vi "Calculate_Release_Flowrates.vi"(3 "Ch names":string[](array[string]), 4 "Units":enum16{"Q l/min", "M_dot Kg/min"}(ring), 5 "Present scan array":dbl[](array[numeric]) format="%.2f") -> (0 "Trace":dbl format="%.2f", 1 "Carrier":dbl format="%.2f", 2 "Scan comments":string)   [LabVIEW 2015]
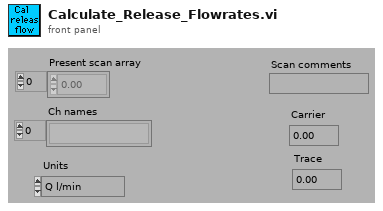
[diagram p1: front panel]
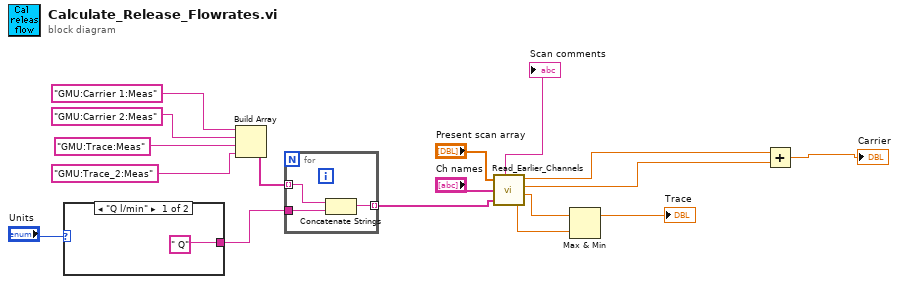
[diagram p0: block diagram]
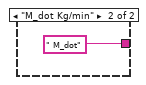
[diagram p2: hidden frame]
diagram:
  n1 = case shown="\"Q l/min\"" "Units" {
    tunnel: [" Q" " M_dot"] -> w16
    frame "Q l/min" {
    }
    frame "M_dot Kg/min" {
    }
  }
  n2 = Build Array("GMU:Carrier 1:Meas", "GMU:Carrier 2:Meas", "GMU:Trace:Meas", "GMU:Trace_2:Meas") -> (w15:string[])
  n3 = for {
    tunnel: w16 -> [w22]
    tunnel: w15 -> [w21] mode=indexing
    tunnel: [w20] -> w7 mode=indexing
    n4 = Concatenate Strings(w21, w22) -> (w20:string)
  }
  n5 = call "Read_Earlier_Channels.vi"("Present scan array"="Present scan array", "Ch names"="Ch names", "Desired Channels"=w7) -> ("Scan comments"=→"Scan comments":string, "Index 0"=w6:dbl, "Index 1"=w5:dbl, "Index 2"=w3:dbl, "Index 3"=w2:dbl)  [unwired: 1 out]
  n6 = Max & Min(x=w3, y=w2) -> (max(x,y)=→"Trace":dbl)  [unwired: 1 out]
  n7 = Add(x=w6, y=w5) -> (x+y=→"Carrier":dbl)
